vi "LVClass_HasoSlopes ctor from has.vi"(0 "HasoSlopes (const)":refnum<class "HasoSlopes.lvclass">, 5 ".has path":path, 11 "error in (no error)":errorcluster) -> (4 "HasoSlopes (new)":refnum<class "HasoSlopes.lvclass">, 15 "error out":errorcluster)   [LabVIEW 2020, in "HasoSlopes.lvclass"]
doc: "HasoSlopes constructor from .has file.\n\n--------------------------------------------------------------------------------\n\n<B>HasoSlopesIn </B> : Constant Pointer to HasoSlopes object.\n<B>HasoSlopesOut </B> : Constant Pointer to HasoSlopes object.\n<B>has_file_path </B> : Absolute path to .has file.\n<B>ErrorIn </B> : Error\n<B>ErrorOut </B> : Error\n\n--------------------------------------------------------------------------------"
uses:
  HasoSlopes.lvclass
  Controls/Handle creation.ctl
  HasoSlopes.lvclass/HasoSlopes.ctl
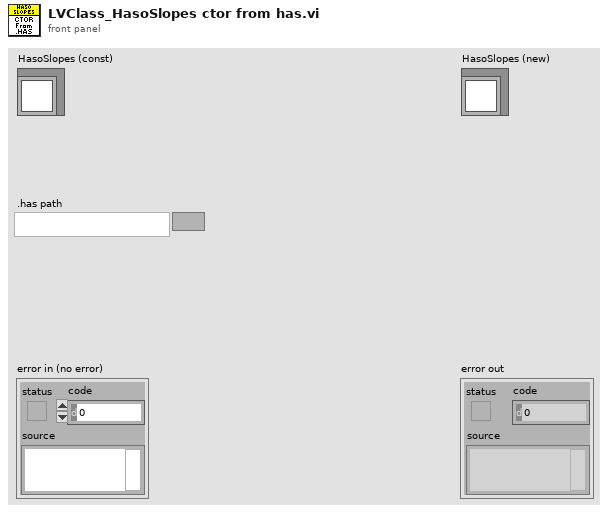
[diagram p1: front panel]
types:
  T1 = typedef "Handle creation.ctl" = enum16{"By ctor", "By write function"}
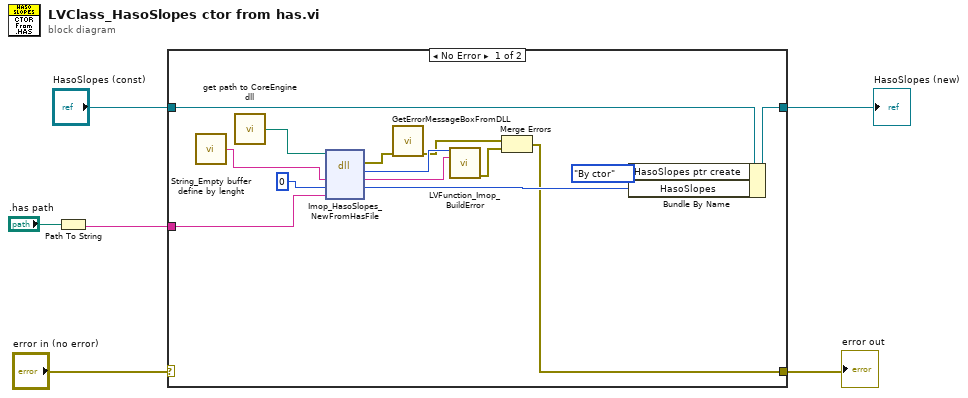
[diagram p0: block diagram]
diagram:
  n1 = Path To String(path=".has path") -> (string=w3:string)
  n2 = case shown="No Error" "error in (no error)" {
    selector: "error in (no error)" -> [_ w22]
    tunnel: [w7 w22] -> w1
    tunnel: [w20 w21] -> w2
    tunnel: "HasoSlopes (const)" -> [w10 w21]
    tunnel: w3 -> [w12 _]
    frame No Error {
      n3 = call "String_Empty buffer define by lenght.vi"() -> ("Empty buffer"=w18:string)  [unwired: 1 in]
      n4 = call "get path to CoreEngine dll.vi"() -> ("path to wavekit library"=w19:path)  [unwired: 14 in, 1 out]
      n5 = dll-call lib="D:/soft/HASO_v3/SVN_trunk/ImOpCoreEngine4_LV2011/DLLs/c_interface_vc100.dll" fn="Imop_HasoSlopes_NewFromHasFile"(path in=w19, "message"=w18, "objet"=0, "chemin_config"=w12) -> (error out=w16:errorcluster, "return type"=w15:i32, "message"=w14:string, "objet"=w13:i64)  [unwired: 3 in, 1 out]
      n6 = call "GetErrorMessageBoxFromDLL.vi"("error IN"=w16) -> ("error OUT"=w9:errorcluster)  [unwired: 10 in]
      n7 = call "LVFunction_Imop_BuildError.vi"("code"=w15, "String to Prepend to source (\"\")"=w14) -> ("error out"=w8:errorcluster)  [unwired: 13 in]
      n8 = Merge Errors(w9, w8) -> (w7:errorcluster)
      n9 = Bundle By Name(cluster=w10, "HasoSlopes ptr create"=Handle_creation."By ctor", "HasoSlopes"=w13) -> (w20:refnum<class "HasoSlopes.lvclass">)
    }
    frame Error {
    }
  }
  "error out" <- w1
  "HasoSlopes (new)" <- w2
